vi "Initialize Locations.vi"(8 "error in":errorcluster, 11 "Save Location":path) -> (0 "error out":errorcluster, 3 "Archivist out":refnum<class "Archivist.lvclass">)   [LabVIEW 2019, in "Archivist.lvclass"]
uses:
  Archivist.lvclass
  Archivist.lvclass/Archivist.ctl
panel:
  in  "Archivist in":refnum<class "Archivist.lvclass">
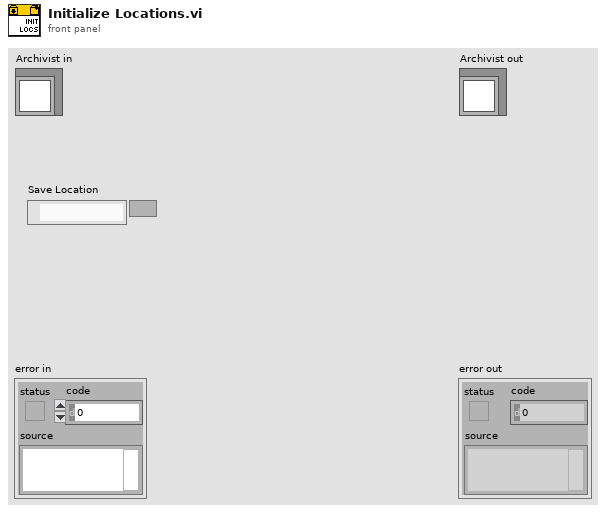
[diagram p1: front panel]
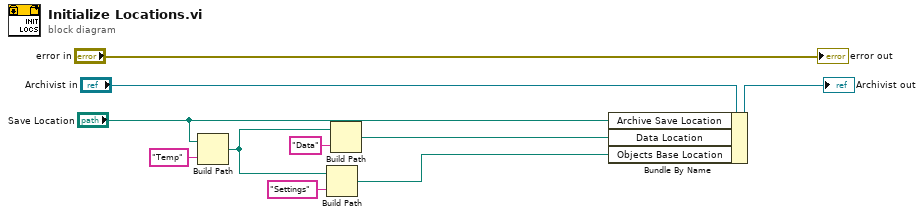
[diagram p0: block diagram]
diagram:
  n1 = Build Path(base path="Save Location", name or relative path="Temp") -> (appended path=w2:path)
  n2 = Build Path(base path=w2, name or relative path="Settings") -> (appended path=w1:path)
  n3 = Build Path(base path=w2, name or relative path="Data") -> (appended path=w4:path)
  n4 = Bundle By Name(cluster="Archivist in", "Archive Save Location"="Save Location", "Data Location"=w4, "Objects Base Location"=w1) -> (→"Archivist out":refnum<class "Archivist.lvclass">)
  "error out" <- "error in"
